vi "NI-DCPower Source DC Voltage.vi"() -> ()   [LabVIEW 2015]
doc: "Demonstrates how to use the DC Voltage Output Function to force an output voltage. This example initializes a session, configures the Output Function, Sense, Autorange, Voltage Level and Current Limit, initiates generation, waits for a specified delay, and measures the voltage and current output. This example uses Single Point source mode."
uses:
  <instrlib>/niDCPower/nidcpower.llb/niDCPower Source Mode.ctl
  <instrlib>/niDCPower/nidcpower.llb/niDCPower Output Function.ctl
  <instrlib>/niDCPower/nidcpower.llb/niDCPower Output State.ctl
  <instrlib>/niDCPower/nidcpower.llb/niDCPower Wait For Event - Event.ctl
panel:
  out "Voltage Measurement 3":dbl caption="Voltage Measurement"
  out "Current Measurement 3":dbl caption="Current Measurement"
  in  "stop":bool
  in  "Source Delay (Sec)":dbl=0.1 format="%_6p"
  out "Voltage Measurement":dbl
  out "Current Measurement":dbl
  in  "Current Limit Range":dbl=0.1 format="%_6p"
  in  "Voltage Level Range":dbl=6.0 format="%_6p"
  out "Compliance/Limit Reached":bool
  in  "Current Limit":dbl=1.0 format="%_6p"
  in  "Voltage Level":dbl=5.0 format="%_6p"
  in  "Channel Name":string="0"
  in  "Resource Name":refnum<k15>="Dev1"
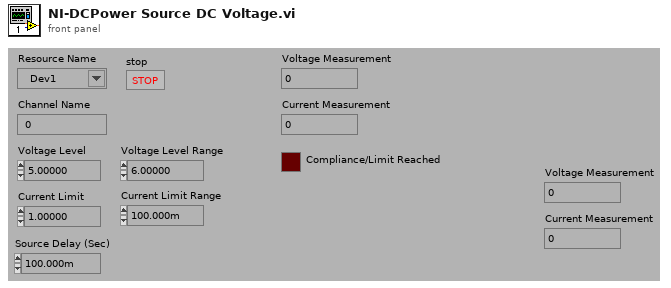
[diagram p1: front panel]
types:
  T1 = typedef "niDCPower Output Function.ctl" = i32
  T2 = typedef "niDCPower Source Mode.ctl" = i32
  T3 = typedef "niDCPower Wait For Event - Event.ctl" = i32
  T4 = typedef "niDCPower Output State.ctl" = u16
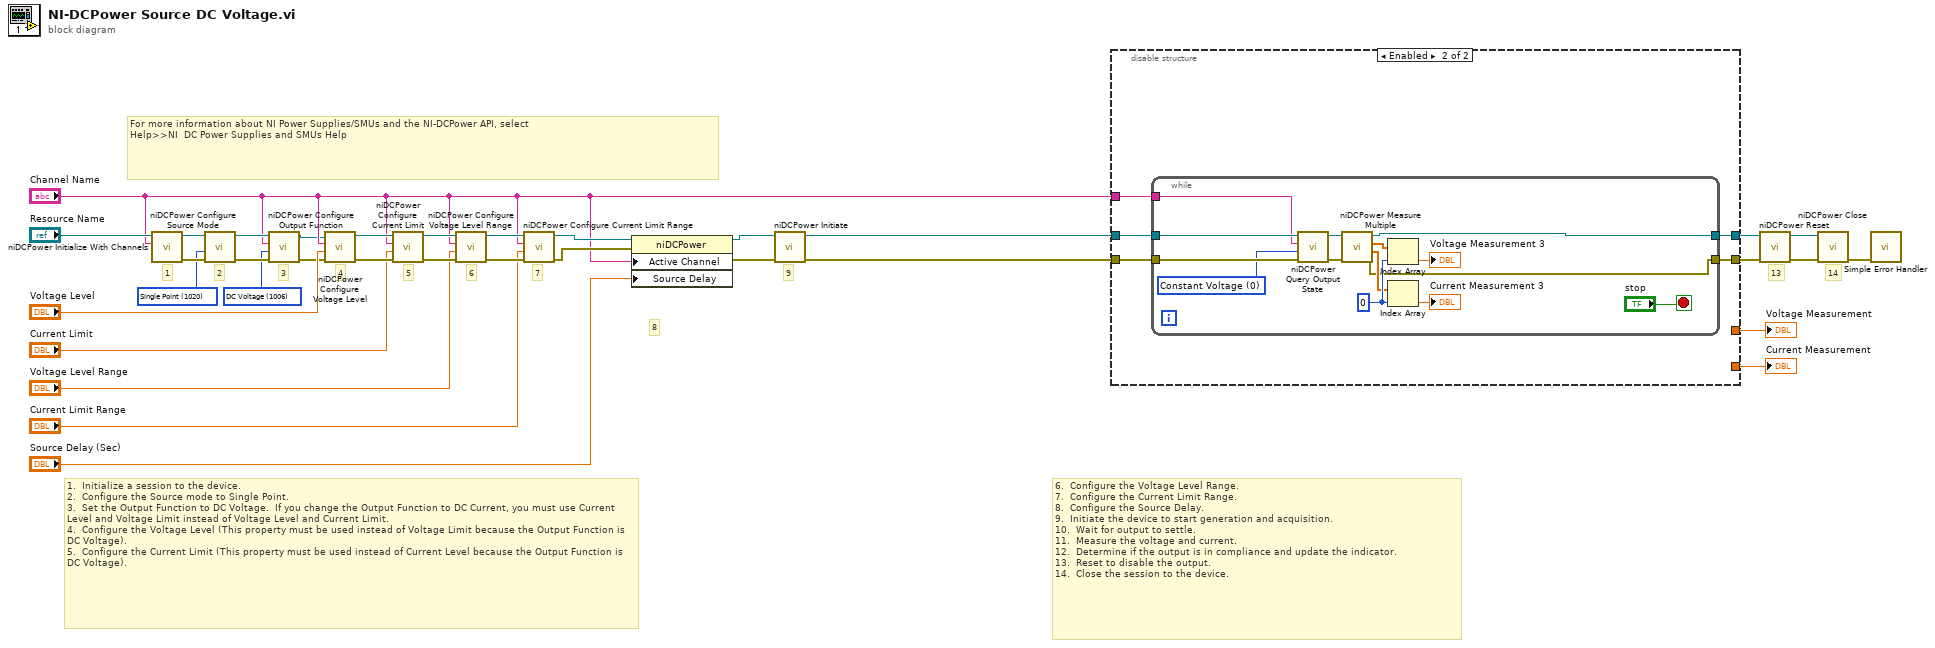
[diagram p0: block diagram]
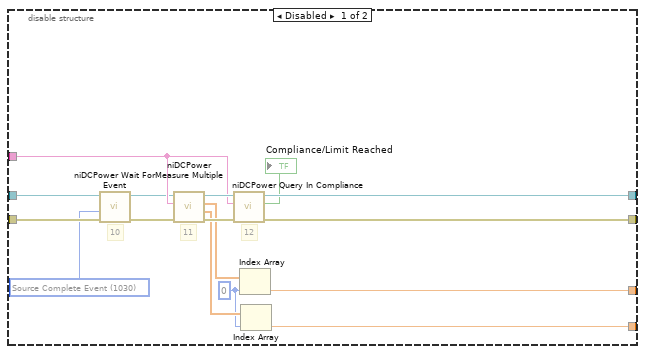
[diagram p2: hidden frame]
diagram:
  w3 = T1 1006 items=["DC Voltage"=1006, "DC Current"=1007, "Pulse Voltage"=1049, "Pulse Current"=1050] ("output function")
  w21 = T2 1020 items=["Single Point"=1020, "Sequence"=1021] ("source mode")
  # "For more information about NI Power Supplies/SMUs and the NI-DCPower API, select\nHelp>>NI  DC Power Supplies and SMUs Help"
  # "14"
  # "9"
  # "7"
  # "6"
  # "2"
  # "1.  Initialize a session to the device.\n2.  Configure the Source mode to Single Point.\n3.  Set the Output Function to DC Voltage.  If you change the Output Function to DC Current, you must use Current Level and Voltage Limit instead of Voltage Level and Current Limit.\n4.  Configure the Voltage Level (This property must be used instead of Voltage Limit because the Output Function is DC Voltage).\n5.  Configure the Current Limit (This property must be used instead of Current Level because the Output Function is DC Voltage)."
  # "3"
  # "6.  Configure the Voltage Level Range.\n7.  Configure the Current Limit Range.\n8.  Configure the Source Delay.\n9.  Initiate the device to start generation and acquisition.\n10.  Wait for output to settle.\n11.  Measure the voltage and current.\n12.  Determine if the output is in compliance and update the indicator.\n13.  Reset to disable the output.\n14.  Close the session to the device."
  # "13"
  # "8"
  # "5"
  # "4"
  # "1"
  n1 = call <instrlib>:"niDCPower Initialize With Channels.vi"("channels"="Channel Name", "resource name"="Resource Name") -> ("error out"=w25:errorcluster, "instrument handle out"=w24:refnum<k15>)  [unwired: 3 in, 5 out]
  n2 = call <instrlib>:"niDCPower Configure Source Mode.vi"("error in (no error)"=w25, "source mode"=w21, "instrument handle"=w24) -> ("error out"=w23:errorcluster, "instrument handle out"=w22:refnum<k15>)  [unwired: 7 out]
  n3 = call <instrlib>:"niDCPower Configure Output Function.vi"("error in (no error)"=w23, "output function"=w3, "channel name"="Channel Name", "instrument handle"=w22) -> ("error out"=w4:errorcluster, "instrument handle out"=w5:refnum<k15>)  [unwired: 6 out]
  n4 = call <instrlib>:"niDCPower Configure Voltage Level.vi"("error in (no error)"=w4, "voltage level"="Voltage Level", "channel name"="Channel Name", "instrument handle"=w5) -> ("error out"=w32:errorcluster, "instrument handle out"=w33:refnum<k15>)  [unwired: 6 out]
  n5 = call <instrlib>:"niDCPower Configure Current Limit.vi"("error in (no error)"=w32, "current limit"="Current Limit", "channel name"="Channel Name", "instrument handle"=w33) -> ("error out"=w20:errorcluster, "instrument handle out"=w19:refnum<k15>)  [unwired: 1 in, 5 out]
  n6 = call <instrlib>:"niDCPower Configure Voltage Level Range.vi"("error in (no error)"=w20, "voltage level range"="Voltage Level Range", "channel name"="Channel Name", "instrument handle"=w19) -> ("error out"=w18:errorcluster, "instrument handle out"=w17:refnum<k15>)  [unwired: 6 out]
  n7 = call <instrlib>:"niDCPower Configure Current Limit Range.vi"("error in (no error)"=w18, "current limit range"="Current Limit Range", "channel name"="Channel Name", "instrument handle"=w17) -> ("error out"=w9:errorcluster, "instrument handle out"=w12:refnum<k15>)  [unwired: 6 out]
  n8 = property class="niDCPower"(reference=w12, error in=w9, "Active Channel"="Channel Name", "Source Delay"="Source Delay (Sec)") -> (reference out=w11:refnum<k15>, error out=w10:errorcluster)
  n9 = call <instrlib>:"niDCPower Initiate.vi"("error in (no error)"=w10, "instrument handle"=w11) -> ("error out"=w6:errorcluster, "instrument handle out"=w1:refnum<k15>)  [unwired: 2 in, 6 out]
  n10 = disable-structure shown="Enabled" {
    disable-tunnel: [w50 w52] -> w30
    disable-tunnel: [w44 _] -> w14
    disable-tunnel: [w43 _] -> w13
    disable-tunnel: "Channel Name" -> [w42 w53]
    disable-tunnel: w1 -> [w41 w55]
    disable-tunnel: w6 -> [w39 w54]
    disable-tunnel: [w35 w51] -> w2
    frame Disabled {
      w37 = T3 1030 items=["Source Complete Event"=1030, "Measure Complete Event"=1031, "Sequence Iteration Complete Event"=1032, "Sequence Engine Done Event"=1033] ("event")
      w45 = 0 ("index")
      # "11"
      # "10"
      # "12"
      n11 = call <instrlib>:"niDCPower Wait For Event.vi"("error in (no error)"=w39, "event"=w37, "instrument handle"=w41) -> ("error out"=w38:errorcluster, "instrument handle out"=w40:refnum<k15>)  [unwired: 1 in, 6 out]
      n12 = call <instrlib>:"niDCPower Measure Multiple.vi"("error in (no error)"=w38, "channel name"=w42, "instrument handle"=w40) -> ("error out"=w48:errorcluster, "current measurements"=w46:dbl[], "voltage measurements"=w47:dbl[], "instrument handle out"=w49:refnum<k15>)  [unwired: 5 out]
      n13 = call <instrlib>:"niDCPower Query In Compliance.vi"("error in (no error)"=w48, "channel name"=w42, "instrument handle"=w49) -> ("error out"=w35:errorcluster, "in compliance?"=→"Compliance/Limit Reached":bool, "instrument handle out"=w50:refnum<k15>)  [unwired: 6 out]
      n14 = Index Array(array=w47, index=w45) -> (element=w43:dbl)
      n15 = Index Array(array=w46, index=w45) -> (element=w44:dbl)
    }
    frame Enabled {
      n16 = while {
        tunnel: w55 -> [w68]
        tunnel: w54 -> [w67]
        tunnel: w53 -> [w66]
        tunnel: [w57] -> w52
        tunnel: [w56] -> w51
        stop <- "stop" stop-if-true
        w64 = 0 ("index")
        w65 = T4 0 items=["Constant Voltage", "Constant Current"] ("output state")
        n17 = call <instrlib>:"niDCPower Query Output State.vi"("error in (no error)"=w67, "output state"=w65, "channel name"=w66, "instrument handle"=w68) -> ("error out"=w59:errorcluster, "instrument handle out"=w58:refnum<k15>)  [unwired: 5 in, 1 out]
        n18 = call <instrlib>:"niDCPower Measure Multiple.vi"("error in (no error)"=w59, "instrument handle"=w58) -> ("error out"=w56:errorcluster, "current measurements"=w60:dbl[], "voltage measurements"=w63:dbl[], "instrument handle out"=w57:refnum<k15>)  [unwired: 1 in, 5 out]
        n19 = Index Array(array=w63, index=w64) -> (element=→"Voltage Measurement 3":dbl)
        n20 = Index Array(array=w60, index=w64) -> (element=→"Current Measurement 3":dbl)
      }
    }
  }
  "Current Measurement" <- w14
  "Voltage Measurement" <- w13
  n21 = call <instrlib>:"niDCPower Reset.vi"("error in (no error)"=w2, "instrument handle"=w30) -> ("error out"=w28:errorcluster, "instrument handle out"=w29:refnum<k15>)  [unwired: 2 in, 6 out]
  n22 = call <instrlib>:"niDCPower Close.vi"("error in (no error)"=w28, "instrument handle"=w29) -> ("error out"=w27:errorcluster)  [unwired: 9 out]
  n23 = call <vilib>:"Simple Error Handler.vi"("error in (no error)"=w27) -> ()  [unwired: 1 in, 8 out]
